vi "Read FIFO.vi"   [LabVIEW 2011, in "FIFO.lvlib"]
uses:
  <instrlib>/RF-RIO/FIFO/FIFO/FPGA/FIFO.lvlib
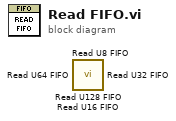
[diagram p0: block diagram]
diagram:
  n1 = call <instrlib>:"Read U128 FIFO.vi"() -> ()  [unwired: 14 in, 2 out]
  n2 = call <instrlib>:"Read U8 FIFO.vi"() -> ()  [unwired: 14 in, 2 out]
  n3 = call <instrlib>:"Read U64 FIFO.vi"() -> ()  [unwired: 14 in, 2 out]
  n4 = call <instrlib>:"Read U32 FIFO.vi"() -> ()  [unwired: 14 in, 2 out]
  n5 = call <instrlib>:"Read U16 FIFO.vi"() -> ()  [unwired: 14 in, 2 out]
